vi "close_driver_session.vi"(5 "Close VISA session (T)":bool=TRUE, 7 "Pause after Close (0)":i32, 8 "error in":errorcluster caption="error in (no error)", 11 "VISA resource name":refnum<visa-resource-name>) -> (0 "error out":errorcluster)   [LabVIEW 2020, in "Rohde&Schwarz RTx Oscilloscopes.lvlib" / "rsidr_core.lvlib"]
uses:
  rsidr_core.lvlib
  _type_Operation_Fgv_Cache.ctl
  _type_Operation_Fgv_RepCap.ctl
  _type_Operation_Fgv_Session.ctl
  _type_Operation_Fgv_Debug.ctl
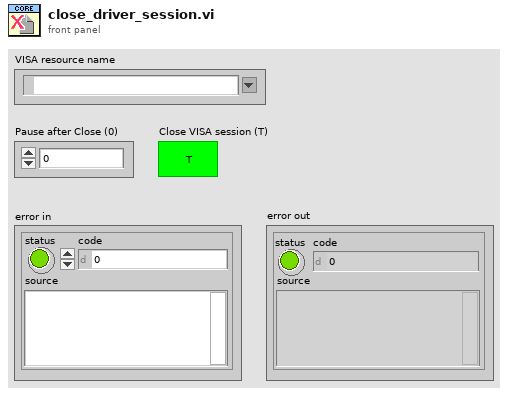
[diagram p1: front panel]
types:
  T1 = typedef "Rohde&Schwarz RTx Oscilloscopes.lvlib/rsidr_core.lvlib/_type_Operation_Fgv_Session.ctl" = enum16{"Initialize", "GetData", "SetData", "Clear", "GetSessionIx"}
  T2 = typedef "Rohde&Schwarz RTx Oscilloscopes.lvlib/rsidr_core.lvlib/_type_Operation_Fgv_RepCap.ctl" = enum16{"Initialize", "Get Cmd Value", "Reset Rep Cap", "Add Rep Cap", "Remove Rep Cap", "Get Rep Cap ID range", "Get Count", "Clear", "Find Name from NameID", "Get First NameID"}
  T3 = typedef "Rohde&Schwarz RTx Oscilloscopes.lvlib/rsidr_core.lvlib/_type_Operation_Fgv_Cache.ctl" = enum16{"Initialize", "Get Cached Value", "Set Cached Value", "Clear"}
  T4 = typedef "Rohde&Schwarz RTx Oscilloscopes.lvlib/rsidr_core.lvlib/type_Session_Data.ctl" = cluster{"IDN string":string, "Instrument FW":string, "Instr type":string, "Instr type for err. msg.":string, "Installed Options":string[], "Ignore Error Messages":string, "Logging params":variant, "OPC Timeout":i32, "VISA Timeout":i32, "STB Poll VISA Timeout":i32, "Additional Flags":i32, "Wait Before Read":i32, "Wait Before Write":i32, "Option String Flags":i32, "IO Segment Size":i64, "VISA Access Mode":T5, "Interface Type":T6, "OPC Wait Mode":T7, "Bin Float Number  Format":T8, "Bin Integer Number Format":T9, "Simulate":bool, "VXIcapable":bool, "Duplicate Session":bool, "Add LF to Write":bool, "Logging":bool, "Fast Sweep":bool, "Query Instrument Status":bool, "Check Range":bool, "Check Options":bool, "OPC-sync Attr Writes":bool, "OPC-sync Attr Queries":bool}
  T5 = typedef "Rohde&Schwarz RTx Oscilloscopes.lvlib/rsidr_core.lvlib/type_VisaAccessMode.ctl" = u16
  T6 = typedef "Rohde&Schwarz RTx Oscilloscopes.lvlib/rsidr_core.lvlib/type_InterfaceType.ctl" = enum16{"Unknown", "GPIB", "VXI", "GPIB_VXI", "ASRL", "PXI", "TCPIP", "USB", "SOCKET"}
  T7 = typedef "Rohde&Schwarz RTx Oscilloscopes.lvlib/rsidr_core.lvlib/type_OPC_Wait_Mode.ctl" = enum16{"STBpolling", "STBpollingSlow", "STBpollingSuperSlow", "ServiceRequest", "OPCquery"}
  T8 = typedef "Rohde&Schwarz RTx Oscilloscopes.lvlib/rsidr_core.lvlib/type_Binary_Float_Number_Format.ctl" = enum16{"Float_4_Bytes_Swapped", "Float_4_Bytes", "Double_8_Bytes_Swapped", "Double_8_Bytes"}
  T9 = typedef "Rohde&Schwarz RTx Oscilloscopes.lvlib/rsidr_core.lvlib/type_Binary_Integer_Number_Format.ctl" = enum16{"Int32_4_Bytes_Swapped", "Int32_4 Bytes", "Int16_2_Bytes_Swapped", "Int16_2_Bytes"}
  T10 = typedef "Rohde&Schwarz RTx Oscilloscopes.lvlib/rsidr_core.lvlib/_type_Operation_Fgv_Debug.ctl" = enum16{"Reset", "ReadCommand", "SetCommand"}
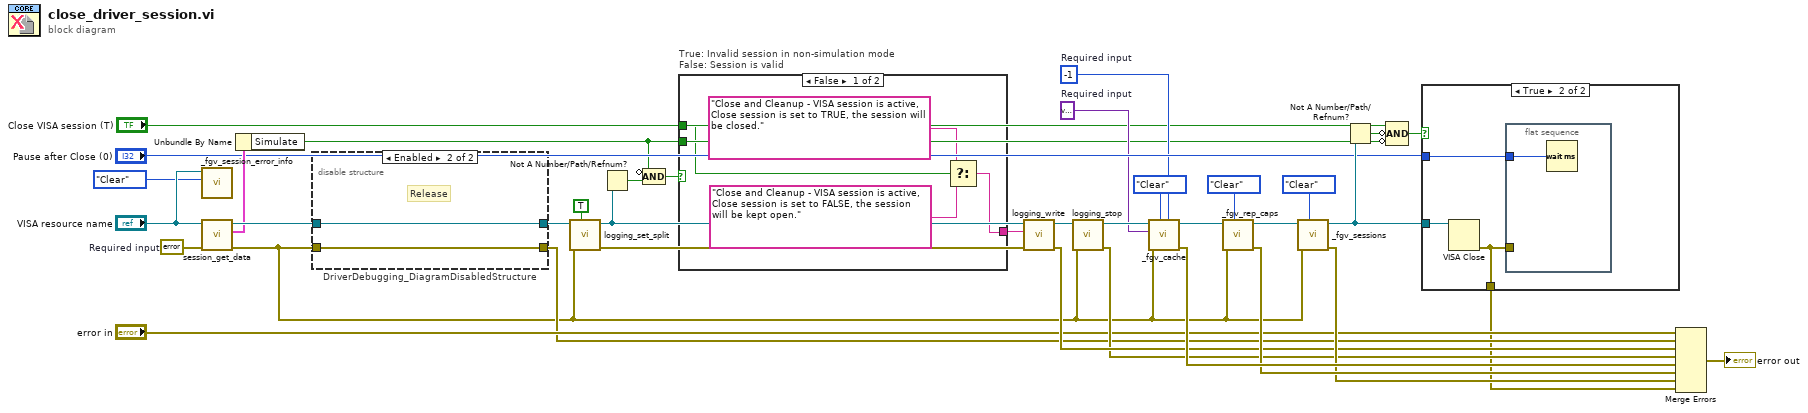
[diagram p0: block diagram]
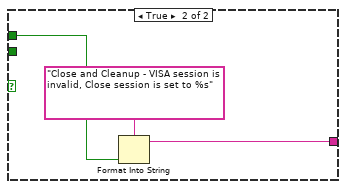
[diagram p2: hidden frame]
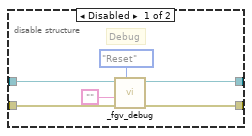
[diagram p3: hidden frame]
diagram:
  w10 = -1  # Required input
  w11 = variant  # Required input
  w20 = errorcluster {"status"=FALSE, "code"=0, "source"=""}  # Required input
  n1 = call "_fgv_session_error_info.vi"("Operation"=_type_Operation_Fgv_Session."Clear", "Session in"="VISA resource name") -> ()  [unwired: 4 in, 2 out]
  n2 = call "session_get_data.vi"("error in"=w20, "VISA resource name"="VISA resource name") -> ("error out"=w19:errorcluster, "Session User Data out"=w18:T4, "VISA resource name out"=w21:refnum<visa-resource-name>)  [unwired: 6 in, 1 out]
  n3 = Unbundle By Name(w18) -> ("Simulate"=w6:bool)
  n4 = disable-structure "DriverDebugging_DiagramDisabledStructure" shown="Enabled" {
    disable-tunnel: w19 -> [w43 w44]
    disable-tunnel: [w41 w44] -> w22
    disable-tunnel: w21 -> [w42 w45]
    disable-tunnel: [w40 w45] -> w24
    frame Disabled {
      # "Debug"
      n5 = call "_fgv_debug.vi"("Operation"=_type_Operation_Fgv_Debug."Reset", "error in"=w43, "Command in"="" ("Empty String Constant"), "VISA resource name"=w42) -> ("error out"=w41:errorcluster, "VISA resource name out"=w40:refnum<visa-resource-name>)  [unwired: 6 in]
    }
    frame Enabled {
      # "Release"
    }
  }
  n6 = call "logging_set_split.vi"("Evaluate section error (F)"=TRUE, "error in"=w19, "VISA resource name"=w24) -> ("error out"=w25:errorcluster, "VISA resource name out"=w9:refnum<visa-resource-name>)  [unwired: 7 in]
  n7 = Not A Number/Path/Refnum?(number/path/refnum=w9) -> (NaN/Path/Refnum?=w7:bool)
  n8 = Compound Arithmetic op=AND(invert w6, w7) -> (w5:bool)
  n9 = case "True: Invalid session in non-simulation mode\nFalse: Session is valid" shown="False" w5 {
    tunnel: [w46 w52] -> w32
    tunnel: "Close VISA session (T)" -> [w49 w50]
    tunnel: w6 -> [_ _]
    frame False {
      n10 = Select(t="Close and Cleanup - VISA session is active, Close session is set to TRUE, the session will be closed." ("String to write"), s=w49, f="Close and Cleanup - VISA session is active, Close session is set to FALSE, the session will be kept open." ("String to write")) -> (s? t:f=w46:string)
    }
    frame True {
      n11 = Format Into String(format string="Close and Cleanup - VISA session is invalid, Close session is set to %s" ("String to write"), w50) -> (resulting string=w52:string)  [unwired: 2 in, 1 out]
    }
  }
  n12 = call "logging_write.vi"("error in"=w25, "String to write"=w32, "VISA resource name"=w9) -> ("error out"=w31:errorcluster, "VISA resource name out"=w27:refnum<visa-resource-name>)  [unwired: 7 in]
  n13 = call "logging_stop.vi"("error in"=w19, "VISA resource name"=w27) -> ("error out"=w30:errorcluster, "VISA resource name out"=w26:refnum<visa-resource-name>)  [unwired: 8 in]
  n14 = call "_fgv_cache.vi"("Index in"=w10, "Operation"=_type_Operation_Fgv_Cache."Clear", "error in"=w19, "Value in"=w11, "VISA resource name"=w26) -> ("error out"=w35:errorcluster, "VISA resource name out"=w37:refnum<visa-resource-name>)  [unwired: 4 in, 1 out]
  n15 = call "_fgv_rep_caps.vi"("Operation"=_type_Operation_Fgv_RepCap."Clear", "error in"=w19, "VISA resource name"=w37) -> ("error out"=w34:errorcluster, "VISA resource name out"=w29:refnum<visa-resource-name>)  [unwired: 5 in, 2 out]
  n16 = call "_fgv_sessions.vi"("Operation"=_type_Operation_Fgv_Session."Clear", "error in"=w19, "VISA resource name"=w29) -> ("error out"=w33:errorcluster, "VISA resource name out"=w28:refnum<visa-resource-name>)  [unwired: 5 in, 2 out]
  n17 = Not A Number/Path/Refnum?(number/path/refnum=w28) -> (NaN/Path/Refnum?=w13:bool)
  n18 = Compound Arithmetic op=AND("Close VISA session (T)", invert w13, invert w6) -> (w12:bool)
  n19 = case shown="True" w12 {
    tunnel: w28 -> [_ w55]
    tunnel: [_ w53] -> w17
    tunnel: "Pause after Close (0)" -> [_ w54]
    frame False {
    }
    frame True {
      n20 = VISA Close(VISA resource name=w55) -> (error out=w53:errorcluster)  [unwired: 1 in]
      n21 = flat-sequence {
        tunnel: w54 -> [w56]
        tunnel: w53 -> [_]
        frame #0 {
          n22 = Wait (ms)(milliseconds to wait=w56) -> ()  [unwired: 1 out]
        }
      }
    }
  }
  n23 = Merge Errors("error in", w22, w31, w30, w35, w34, w33, w17) -> (→"error out":errorcluster)
